vi "MakeZeroIfNegative.vi"(1 "Number":dbl) -> (0 "Result":dbl)   [LabVIEW 2009]
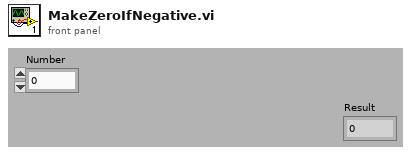
[diagram p1: front panel]
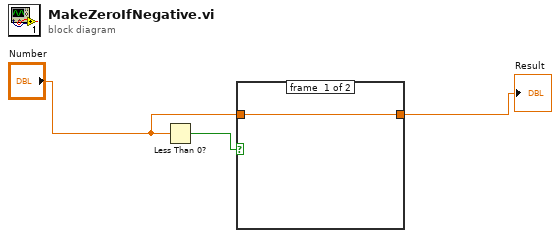
[diagram p0: block diagram]
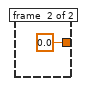
[diagram p2: hidden frame]
diagram:
  n1 = Less Than 0?(x="Number") -> (x < 0?=w3:bool)
  n2 = case shown="True" w3 {
    tunnel: [w4 0.0 ("Number")] -> w2
    tunnel: "Number" -> [w4 _]
    frame #0 {
    }
    frame #1 {
    }
  }
  "Result" <- w2
